vi "LMS_SetSampleRate.vi"(8 "error in (no error)":errorcluster, 9 "oversample":u64, 10 "rate":dbl, 11 "device_In":i64) -> (0 "error out":errorcluster, 3 "device_Out":i64)   [LabVIEW 2013, in "LMS_LV_Drv.lvlib"]
uses:
  LMS_LV_Drv.lvlib
  LimeSuite.dll
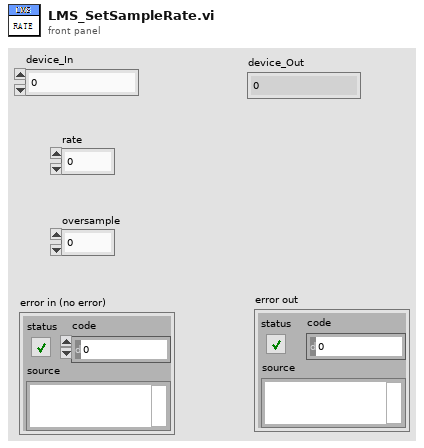
[diagram p1: front panel]
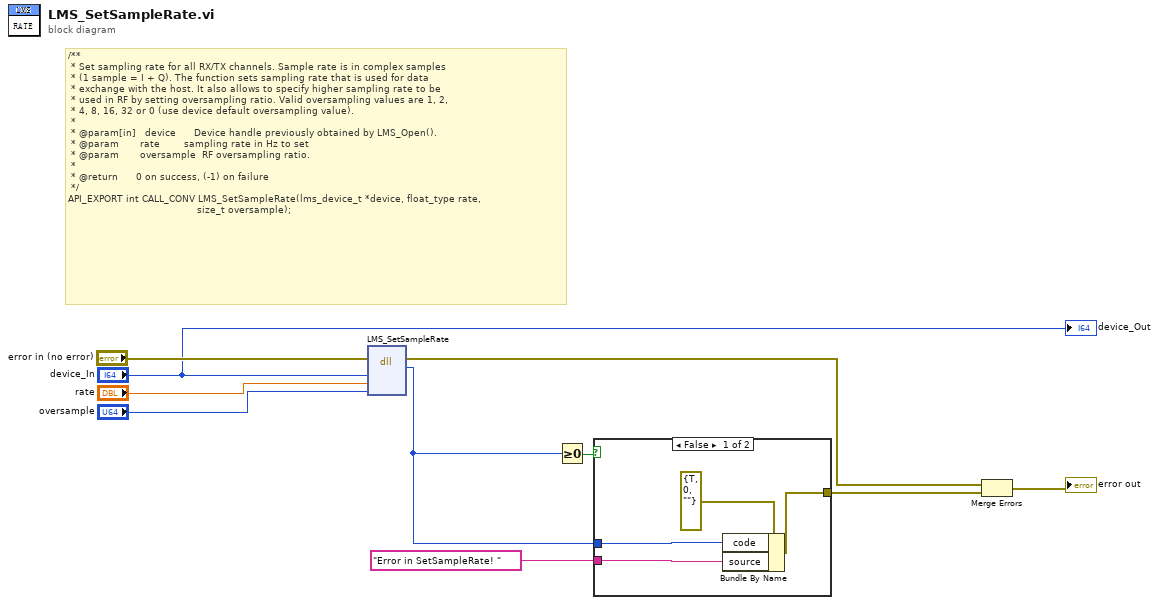
[diagram p0: block diagram]
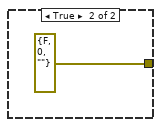
[diagram p2: hidden frame]
diagram:
  # "/**\n * Set sampling rate for all RX/TX channels. Sample rate is in complex samples\n * (1 sample = I + Q). The function sets sampling rate that is used for data\n * exchange with the host. It also allows to specify higher sampling rate to be\n * used in RF by setting oversampling ratio. Valid oversampling values are 1, 2,\n * 4, 8, 16, 32 or 0 (use device default oversampling value).\n *\n * @param[in]   device      Device handle previously obtained by LMS_Open().\n * @param       rate        sampling rate in Hz to set\n * @param       oversample  RF oversampling ratio.\n *\n * @return      0 on success, (-1) on failure\n */\nAPI_EXPORT int CALL_CONV LMS_SetSampleRate(lms_device_t *device, float_type rate,\n                                           size_t oversample);"
  n1 = dll-call lib="PTH1mabs CUsersOTADesktop书籍出版程序8.第八章LimeSDR_LabVIEW_Driver-master\nLimeSuite.dll" fn="LMS_SetSampleRate"(error in="error in (no error)", "device"="device_In", "rate"="rate", "oversample"="oversample") -> (error out=w2:errorcluster, "return type"=w3:i32)  [unwired: 5 in, 1 out]
  n2 = Greater Or Equal To 0?(x=w3) -> (x >= 0?=w6:bool)
  n3 = case shown="False" w6 {
    tunnel: [w13 errorcluster {"status"=FALSE, "code"=0, "source"=""} ("error in")] -> w4
    tunnel: w3 -> [w12 _]
    tunnel: "Error in SetSampleRate! " ("source") -> [w11 _]
    frame False {
      n4 = Bundle By Name(cluster=errorcluster {"status"=TRUE, "code"=0, "source"=""} ("error in"), "code"=w12, "source"=w11) -> (w13:errorcluster)
    }
    frame True {
    }
  }
  n5 = Merge Errors(w2, w4) -> (→"error out":errorcluster)
  "device_Out" <- "device_In"
